vi "Write Version String.vi"(8 "error in (no error)":errorcluster, 10 "Version String":string, 11 "LabVIEW File in":refnum<class "LabVIEW File.lvclass">) -> (0 "error out":errorcluster, 3 "LabVIEW File out":refnum<class "LabVIEW File.lvclass">)   [LabVIEW 2020, in "Save for Previous Version.lvlib" / "LabVIEW File.lvclass"]
uses:
  LabVIEW File.lvclass
  LabVIEW File.lvclass/LabVIEW File.ctl
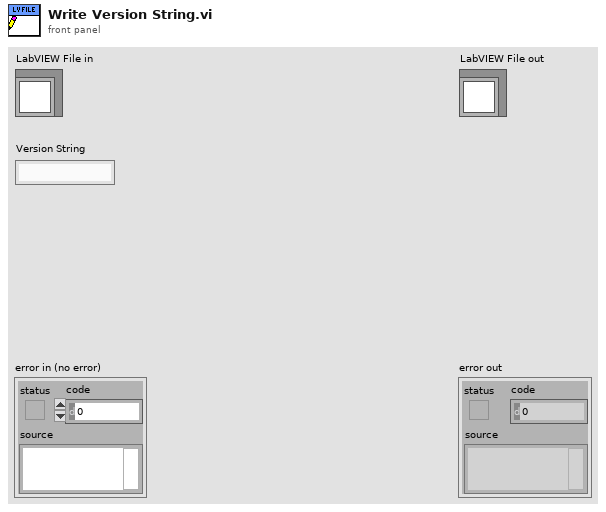
[diagram p1: front panel]
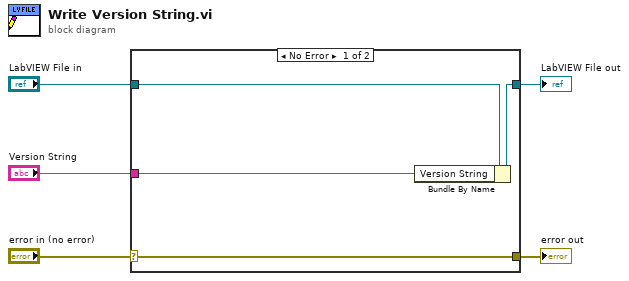
[diagram p0: block diagram]
diagram:
  n1 = case shown="No Error" "error in (no error)" {
    selector: "error in (no error)" -> [w9 w10]
    tunnel: [w9 w10] -> w4
    tunnel: [w7 w11] -> w2
    tunnel: "LabVIEW File in" -> [w8 w11]
    tunnel: "Version String" -> [w6 _]
    frame No Error {
      n2 = Bundle By Name(cluster=w8, "Version String"=w6) -> (w7:refnum<class "LabVIEW File.lvclass">)
    }
    frame Error {
    }
  }
  "error out" <- w4
  "LabVIEW File out" <- w2
